vi "GEM_BANK_IsNameMatch.vi"(8 "error in (no error)":errorcluster, 10 "GEM_BANK Cluster":T1, 11 "LVBANK in":refnum<class "GEM_BANK.lvclass">) -> (0 "error out":errorcluster, 2 "BANK MATCHES":bool, 3 "LVBANK out":refnum<class "GEM_BANK.lvclass">)   [LabVIEW 2018, in "GEM_BANK.lvclass"]
uses:
  GEM_BANK.lvclass
  GEM_BANK_CLUSTER_typedef.ctl
  GEM_DATA_cluster_typedef.ctl
  GEM_BANK.lvclass/GEM_BANK.ctl
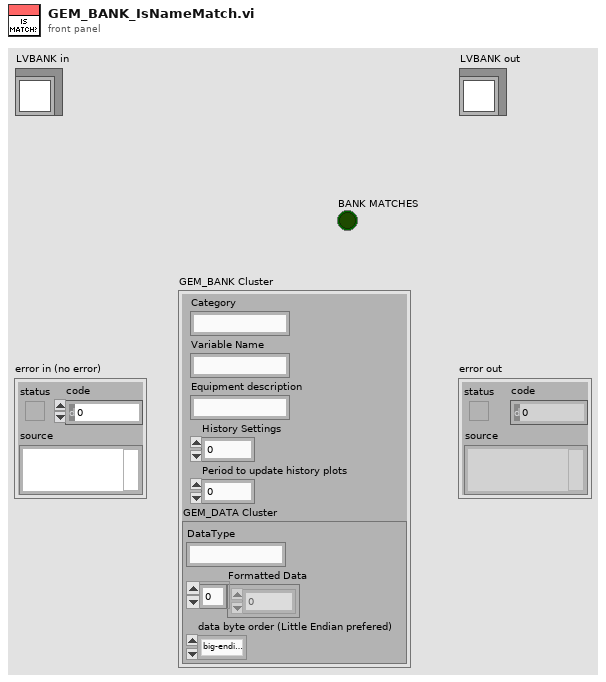
[diagram p1: front panel]
types:
  T1 = typedef "GEM_BANK_CLUSTER_typedef.ctl" = cluster{"Category":string, "Variable Name":string, "Equipment description":string, "History Settings":u16, "Period to update history plots":u16, "GEM_DATA Cluster":T2}
  T2 = typedef "GEM_DATA_cluster_typedef.ctl" = cluster{"DataType":string, "Formatted Data":u8[], "data byte order (Little Endian prefered)":enum16{"big-endian, network order", "native, host order", "little-endian"}}
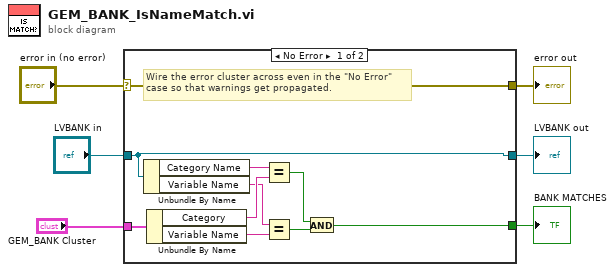
[diagram p0: block diagram]
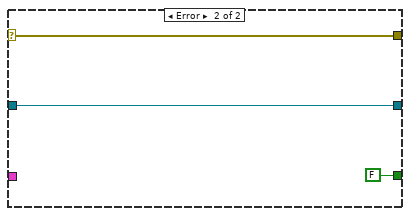
[diagram p2: hidden frame]
diagram:
  n1 = case shown="No Error" "error in (no error)" {
    selector: "error in (no error)" -> [w16 w19]
    tunnel: [w16 w19] -> w5
    tunnel: [w15 w18] -> w3
    tunnel: "LVBANK in" -> [w15 w18]
    tunnel: [w7 FALSE] -> w2
    tunnel: "GEM_BANK Cluster" -> [w14 _]
    frame No Error {
      # "Wire the error cluster across even in the \"No Error\"\ncase so that warnings get propagated."
      n2 = Unbundle By Name(w15) -> ("Category Name"=w13:string, "Variable Name"=w10:string)
      n3 = Unbundle By Name(w14) -> ("Category"=w12:string, "Variable Name"=w9:string)
      n4 = Equal?(x=w13, y=w12) -> (x = y?=w11:bool)
      n5 = Equal?(x=w10, y=w9) -> (x = y?=w8:bool)
      n6 = And(x=w11, y=w8) -> (x .and. y?=w7:bool)
    }
    frame Error {
    }
  }
  "error out" <- w5
  "LVBANK out" <- w3
  "BANK MATCHES" <- w2
